vi "Stimulus trigger period event handler.vi"   [LabVIEW 2013]
uses:
  Global Variables/FPGAstatus_Reference.vi
  Global Variables/gl_UI Ctrl Refs.vi
types:
  T1 = typedef "UI ctrl refs cluster.ctl" = cluster{"Top level VI path":path, "Top level VI ref":refnum<vi>, "User menu ref":refnum<k9>, "Sub Panel control":refnum<vi>, "Imaging Param Tab":refnum<vi>, "Occurrence-Start drivers":refnum<k4>, "Occurrence-Speed logging initialised":refnum<k4>, "Occurrence-XYZ stage initialised":refnum<k4>, "Exit button":refnum<vi>, "Status ind":refnum<vi>, "Return to Origin":refnum<vi>, "Speed Logging":refnum<vi>, "Time Lapse":refnum<vi>, "Live Imaging":refnum<vi>, "AOL Z Stack":refnum<vi>, "Motor Z Stack":refnum<vi>, "Funct Acq button":refnum<vi>, "Hard Shutter":refnum<vi>, "Virtual Shutter":refnum<vi>, "Laser Power":refnum<vi>, "AOL Mode":refnum<vi>, "Frame Size":refnum<vi>, "Field of View":refnum<vi>, "Dwell Time":refnum<vi>, "Zoom":refnum<vi>, "AOL Z":refnum<vi>, "Objective":refnum<vi>, "Axis":refnum<vi>, "Paths & Names":refnum<vi>, "Experiment folder path (ind.)":refnum<vi>, "Last State (Ind.)":refnum<vi>, "Laser wavelength ind (nm)":refnum<vi>, "Averages":refnum<vi>, "Angle (degrees)":refnum<vi>, "X centre":refnum<vi>, "Y centre":refnum<vi>, "Plane Mode":refnum<vi>, "# Planes":refnum<vi>, "Z Start":refnum<vi>, "Z Stop":refnum<vi>, "Z Step":refnum<vi>, "PMT 1":refnum<vi>, "PMT 2":refnum<vi>, "Stage XYZ Position":refnum<vi>, "Pockels@Z Start":refnum<vi>, "Pockels@Z Stop":refnum<vi>, "Obtain Z Start":refnum<vi>, "Obtain Z Stop":refnum<vi>, "Live stim.trig.period":refnum<vi>, "Live stim.trig.enable":refnum<vi>, "Funct. Acq. Pockels Modulation":refnum<vi>, "Enable Video Recording":refnum<vi>, "Video Record-Live Imaging":refnum<vi>, "Video Record-Funct acq":refnum<vi>, "AOL Z-stack Chirps Ready (ind)":refnum<vi>, "Center freq ind (nm)":refnum<vi>, "Logging queue (ind)":refnum<vi>, "Back aperture power (ind.)":refnum<vi>, "Power after objective (ind.)":refnum<vi>, "Switch user":refnum<vi>}
  T2 = typedef "FPGA Ref.ctl" = refnum<k20>
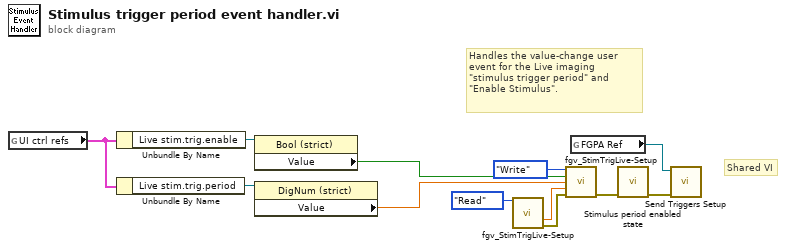
[diagram p0: block diagram]
diagram:
  # "Shared VI"
  # "Handles the value-change user event for the Live imaging \"stimulus trigger period\" and \"Enable Stimulus\"."
  n1 = global read "gl_UI Ctrl Refs.vi" "UI ctrl refs"() -> (w5:T1)
  n2 = Unbundle By Name(w5) -> ("Live stim.trig.enable"=w10:refnum<vi>)
  n3 = Unbundle By Name(w5) -> ("Live stim.trig.period"=w9:refnum<vi>)
  n4 = property on="Property Node" class="Bool (strict)"(reference=w10) -> ("Value"=w7:bool)  [unwired: 1 in, 2 out]
  n5 = property on="Property Node" class="DigNum (strict)"(reference=w9) -> ("Value"=w6:dbl)  [unwired: 1 in, 2 out]
  n6 = call "fgv_StimTrigLive-Setup.vi"("Function"=enum16{"Intialize", "Write", "Read", "Clear"}."Read") -> ("Live stim.trig.width (ms)"=w1:dbl, "error out"=w2:errorcluster)  [unwired: 11 in, 2 out]
  n7 = call "fgv_StimTrigLive-Setup.vi"("Function"=enum16{"Intialize", "Write", "Read", "Clear"}."Write", "Live stim.trig.enable"=w7, "Live stim.trig.period (sec)"=w6, "Live stim.trig.width (ms)"=w1, "error in (no error)"=w2) -> ("error out"=w4:errorcluster)  [unwired: 7 in, 3 out]
  n8 = global read "FPGAstatus_Reference.vi" "FGPA Ref"() -> (w12:T2)
  n9 = call "Stimulus period enabled state.vi"("error in (no error)"=w4) -> ("error out"=w11:errorcluster)  [unwired: 10 in]
  n10 = call "Send Triggers Setup.vi"("error in (no error)"=w11, "FGPA Ref"=w12) -> ()  [unwired: 8 in, 2 out]
